vi "Create User Event - Stop.vi"(8 "error in (no error)":T1 caption="entrée d'erreur (pas d'erreur)") -> (0 "error out":T1 caption="sortie d'erreur", 2 "Événement utilisateur - Arrêt":refnum<user-event>, 3 "Refnum Enregistrement à l'événement Arrêt":refnum<event-registration>)   [LabVIEW 2012, in "User Event - Stop.lvlib"]
doc: "Créer un événement utilisateur booléen qui sera utilisé pour arrêter la boucle d'événement à partir de la boucle de gestion de messages."
uses:
  User Event - Stop.lvlib
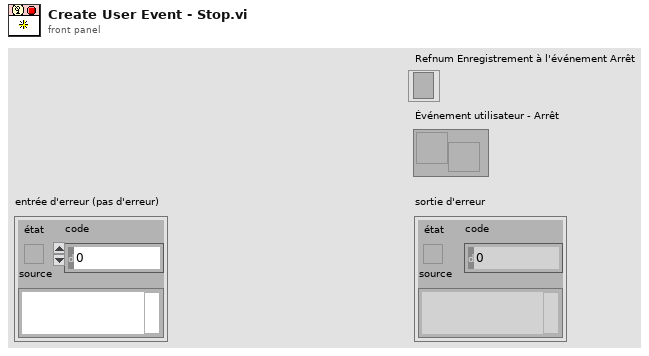
[diagram p1: front panel]
types:
  T1 = cluster{"état":bool, "code":i32, "source":string}
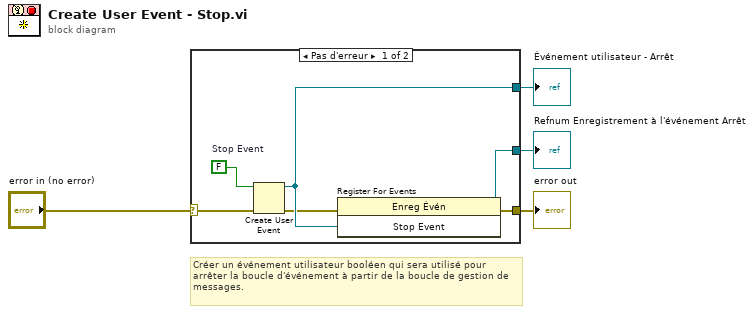
[diagram p0: block diagram]
diagram:
  # "Créer un événement utilisateur booléen qui sera utilisé pour arrêter la boucle d'événement à partir de la boucle de gestion de messages."
  n1 = case shown="Pas d'erreur" "error in (no error)" {
    selector: "error in (no error)" -> [w5 w11]
    tunnel: [w10 _] -> w4
    tunnel: [w9 _] -> w3
    tunnel: [w6 w11] -> w2
    frame No Error {
      w8 = FALSE  # Stop Event
      n2 = Create User Event(user event datatype=w8, error in=w5) -> (user event=w10:refnum<user-event>, error out=w7:errorcluster)
      n3 = register-events(error in=w7, w10) -> (reference out=w9:refnum<event-registration>, error out=w6:errorcluster)  [unwired: 1 in]
    }
    frame Error {
    }
  }
  "Événement utilisateur - Arrêt" <- w4
  "error out" <- w2
  "Refnum Enregistrement à l'événement Arrêt" <- w3
